vi "connection_process.vi"(6 "timeout (ms)":i32=1000, 11 "Connection":refnum<class "Connection.lvclass">) -> ()   [LabVIEW 2013, in "Connection_GOSPL.lvlib" / "Connection.lvclass"]
uses:
  Connection.lvclass
  Connection.lvclass/Connection.ctl
  reason -- ring.ctl
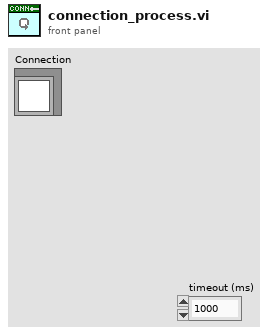
[diagram p1: front panel]
types:
  T1 = typedef "Connection_GOSPL.lvlib/Connection.lvclass/reason -- ring.ctl" = u16
  T2 = cluster{"Connection out":refnum<class "Connection.lvclass">, "error out":errorcluster}
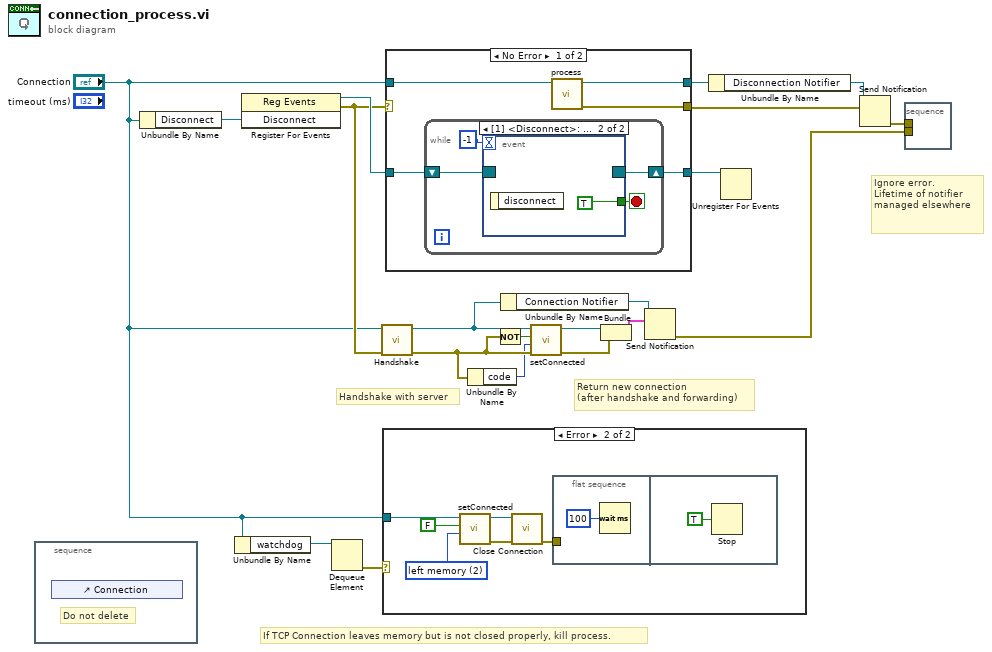
[diagram p0: block diagram]
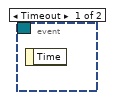
[diagram p3: hidden frame]
diagram:
  # "Return new connection\n(after handshake and forwarding)"
  # "Handshake with server"
  # "If TCP Connection leaves memory but is not closed properly, kill process."
  # "Ignore error.\nLifetime of notifier managed elsewhere"
  n1 = stacked-sequence {
    frame #0 {
      # "Do not delete"
      n2 = control-ref of="Connection"() -> ()  [unwired: 1 out]
    }
  }
  n3 = Unbundle By Name("Connection") -> ("Disconnect"=w17:refnum<user-event>)
  n4 = Unbundle By Name("Connection") -> ("watchdog"=w15:refnum<queue>)
  n5 = register-events(w17) -> (reference out=w18:refnum<event-registration>, error out=w13:errorcluster)  [unwired: 2 in]
  n6 = Dequeue Element(queue=w15) -> (error out=w14:errorcluster)  [unwired: 2 in, 3 out]
  n7 = call-dynamic "Handshake.vi"("error in (no error)"=w13, "Connection in"="Connection") -> ("error out"=w2:errorcluster, "Connection out"=w6:refnum<class "Connection.lvclass">)  [unwired: 8 in]
  n8 = case shown="Error" w14 {
    tunnel: "Connection" -> [_ w25]
    frame No Error {
    }
    frame Error {
      w21 = T1 2 items=["nominal"=0, "unspecified"=1, "left memory"=2, "timed out"=56, "disconnected by peer"=66] ("Reason")
      n9 = call "setConnected.vi"("reason"=w21, "connected"=FALSE, "Connection in"=w25) -> ("error out"=w23:errorcluster, "Connection out"=w24:refnum<class "Connection.lvclass">)  [unwired: 7 in]
      n10 = call "Close Connection.vi"("error in (no error)"=w23, "Connection in"=w24) -> ("error out"=w26:errorcluster)  [unwired: 8 in, 1 out]
      n11 = flat-sequence {
        tunnel: w26 -> [_]
        frame #0 {
          n12 = Wait (ms)(milliseconds to wait=u32 100) -> ()  [unwired: 1 out]
        }
        frame #1 {
          n13 = Stop(stop? (T)=TRUE) -> ()
        }
      }
    }
  }
  n14 = case shown="No Error" w13 {
    selector: w13 -> [_ w40]
    tunnel: [w33 w41] -> w19
    tunnel: w18 -> [w32 w41]
    tunnel: [w30 w40] -> w16
    tunnel: "Connection" -> [w31 w39]
    tunnel: [w29 w39] -> w8
    frame No Error {
      n15 = while {
        shift-right: [w36] -> w33
        shift-left: w32 -> [w35]
        stop <- w34 stop-if-true
        n16 = event shown="[1] <Disconnect>: User Event" {
          selector: w35 -> [_ _]
          dyn-events: [_ _] -> w36
          timeout: -1 -> [_ _]
          tunnel: [_ TRUE] -> w34
          event Timeout {
            n17 = event-data() -> ()  [unwired: 1 in, 1 out]
          }
          event User Event {
            n18 = event-data() -> ()  [unwired: 1 in, 1 out]
          }
        }
      }
      n19 = call-dynamic "process.vi"("Connection in"=w31) -> ("error out"=w30:errorcluster, "Connection out"=w29:refnum<class "Connection.lvclass">)  [unwired: 9 in]
    }
    frame Error {
    }
  }
  n20 = Unbundle By Name(w2) -> ("code"=w1:i32)
  n21 = Not(x=w2) -> (.not. x?=w9:bool)
  n22 = Unbundle By Name(w6) -> ("Connection Notifier"=w5:refnum<notifier>)
  n23 = call "setConnected.vi"("error in (no error)"=w2, "reason"=w1, "connected"=w9, "Connection in"=w6) -> ("error out"=w11:errorcluster, "Connection out"=w10:refnum<class "Connection.lvclass">)  [unwired: 6 in]
  n24 = Bundle("Connection out"=w10, "error out"=w11) -> (w20:T2)  [unwired: 1 in]
  n25 = Send Notification(notification=w20, notifier=w5) -> (error out=w3:errorcluster)  [unwired: 1 in, 1 out]
  n26 = Unbundle By Name(w8) -> ("Disconnection Notifier"=w7:refnum<notifier>)
  n27 = Unregister For Events(event registration refnum=w19) -> ()  [unwired: 1 in, 1 out]
  n28 = Send Notification(notification=w16, notifier=w7) -> (error out=w12:errorcluster)  [unwired: 1 in, 1 out]
  n29 = stacked-sequence {
    tunnel: w12 -> [_]
    tunnel: w3 -> [_]
    frame #0 {
    }
  }
